vi "tm481_wview_wVision.vi"() -> ()   [LabVIEW 2021]
panel:
  out "Display":T1(plugin-control)
  in  "Vertical Width":i32=512
  in  "Horizontal Width":i32=512
  in  "Vertical Offset B":i32=64
  in  "Horizontal Offset B":i32=256
  in  "Vertical Offset A":i32=128
  in  "Horizontal Offset A":i32=512
  out "Frames Per Second":dbl
  in  "Quit":bool
  out "Error Out":errorcluster {"code" format="%.0x"}
  # "This is just a simple example\nof how to setup a camera for\na W-View application with\na Flash4.0 LT"
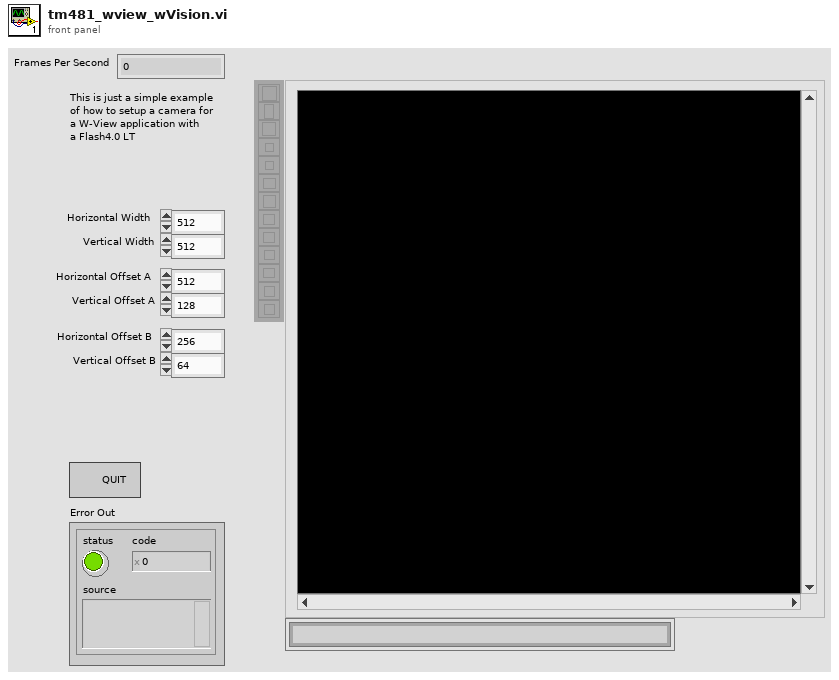
[diagram p1: front panel]
types:
  T1 = typedef "IMAQ Image.ctl" = refnum<image>
  T2 = typedef "Image Type" = u32
  T3 = cluster{"Horizontal Offset A":i32, "Vertical Offset A":i32, "Horizontal Offset B":i32, "Vertical Offset B":i32, "Horizontal Width":i32, "Vertical Width":i32}
  T4 = cluster{"height":i32, "width":i32, "datatype":i32}
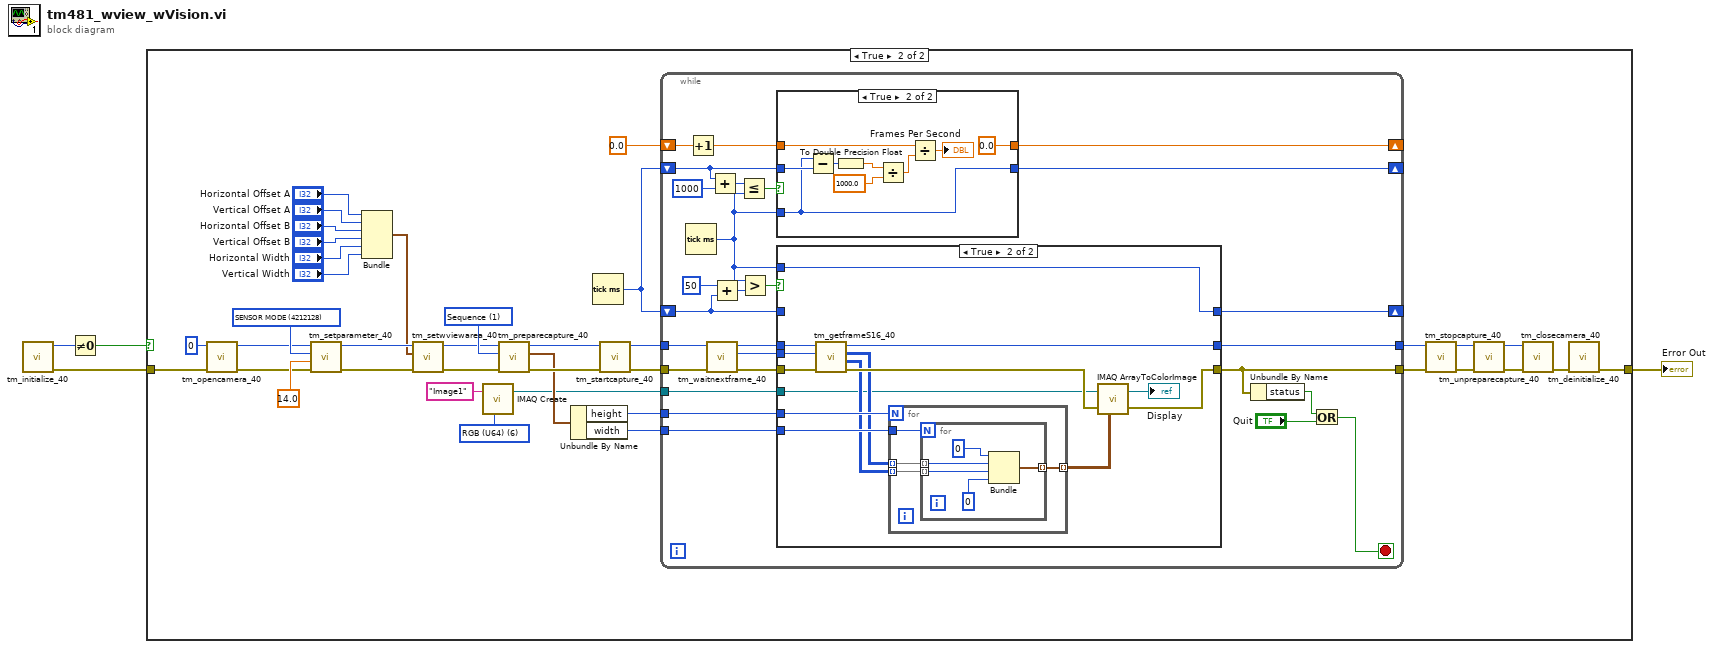
[diagram p0: block diagram]
diagram:
  n1 = call <userlib>:"tm_initialize_40.vi"() -> ("error out"=w1:errorcluster, "Number Of Cameras"=w2:u32)  [unwired: 8 in, 2 out]
  n2 = Not Equal To 0?(x=w2) -> (x != 0?=w4:bool)
  n3 = case shown="True" w4 {
    tunnel: w1 -> [w5 w43]
    tunnel: [w5 w40] -> w3
    frame False {
    }
    frame True {
      w9 = T2 6 items=["Grayscale (U8)", "Grayscale (I16)", "Grayscale (SGL)", "Complex (CSG)", "RGB (U32)", "HSL (U32)", "RGB (U64)", "Grayscale (U16)"] ("Image Type")
      w25 = u32 4212128 items=["SENSOR MODE"=4212128, "CCD MODE"=4212384, "READOUT MODE"=4211872, "ACTIVE VIEW INDEX"=4343136, "BITS PER CHANNEL"=4342976, "IMAGE PIXEL TYPE"=4343296, "BINNING"=4215968, "EXPOSURE TIME"=2049184, "CONTRAST GAIN"=3163312, "CONTRAST OFFSET"=3163328, "LIGHT MODE"=2114720, "SENSITIVITY"=2114992, "PHOTON IMAGING MODE"=2115200, "HIGH DYNAMIC RANGE MODE"=3163360, "WHITE BALANCE"=3163568, "TEMPERATURE"=2115232, "TEMPERATURE TARGET"=2115264, "SENSOR COOLER FAN"=2115296, "LINEBUNDLE HEIGHT"=4212192, "MECHANICAL SHUTTER"=2115488, "BACK FOCUS POSITION"=8422304, "TRIGGER CONNECTOR"=1066432, "TRIGGER SOURCE"=1066144, "OUTPUT TRIGGER SOURCE"=1852576, "TRIGGER GLOBAL EXPOSURE"=2049680, "FIRST TRIGGER BEHAVIOR"=2049696, "CHANNEL SYNC"=1852352, "READOUT DIRECTION"=4211904, "PRE HSYNC COUNT"=1852704, "INTERNAL LINE SPEED"=4191408, "INTERNAL LINE INTERVAL"=4191424] ("Parameter")
      w31 = 1 items=["Snap", "Sequence"] ("Capture mode")
      n4 = call <userlib>:"tm_opencamera_40.vi"("error in (no error)"=w43, "Camera Index"=u32 0) -> ("error out"=w23:errorcluster, "Handle out"=w24:u32)  [unwired: 7 in, 1 out]
      n5 = call <userlib>:"tm_setparameter_40.vi"("error in (no error)"=w23, "Value in"=14.0, "Parameter"=w25, "Handle in"=w24) -> ("error out"=w21:errorcluster, "Handle out"=w22:u32)  [unwired: 6 in]
      n6 = Bundle("Horizontal Offset A"="Horizontal Offset A", "Vertical Offset A"="Vertical Offset A", "Horizontal Offset B"="Horizontal Offset B", "Vertical Offset B"="Vertical Offset B", "Horizontal Width"="Horizontal Width", "Vertical Width"="Vertical Width") -> (w18:T3)  [unwired: 1 in]
      n7 = call <userlib>:"tm_setwviewarea_40.vi"("error in (no error)"=w21, "Sub Region"=w18, "Handle in"=w22) -> ("error out"=w20:errorcluster, "Handle out"=w19:u32)  [unwired: 7 in]
      n8 = call "IMAQ Create"("Image Name"="Image1", "Image Type"=w9) -> ("New Image"=w8:T1)  [unwired: 3 in, 1 out]
      n9 = call <userlib>:"tm_preparecapture_40.vi"("error in (no error)"=w20, "Capture mode"=w31, "Handle in"=w19) -> ("error out"=w29:errorcluster, "Buffer Info"=w11:T4, "Handle out"=w30:u32)  [unwired: 5 in, 1 out]
      n10 = Unbundle By Name(w11) -> ("height"=w7:i32, "width"=w6:i32)
      n11 = Tick Count (ms)() -> (millisecond timer value=w27:u32)
      n12 = call <userlib>:"tm_startcapture_40.vi"("error in (no error)"=w29, "Handle in"=w30) -> ("error out"=w32:errorcluster, "Handle out"=w33:u32)  [unwired: 8 in]
      n13 = while {
        tunnel: [w49] -> w36
        tunnel: [w50] -> w37
        tunnel: w33 -> [w67]
        tunnel: w32 -> [w68]
        shift-right: [w65] -> _
        shift-left: w27 -> [w62]
        shift-right: [w66] -> _
        shift-left: 0.0 -> [w59]
        shift-right: [w48] -> _
        shift-left: w27 -> [w51]
        tunnel: w7 -> [w47]
        tunnel: w6 -> [w46]
        tunnel: w8 -> [w45]
        stop <- w44 stop-if-true
        n14 = Tick Count (ms)() -> (millisecond timer value=w52:u32)
        n15 = Increment(x=w59) -> (x+1=w60:dbl)
        n16 = call <userlib>:"tm_waitnextframe_40.vi"("error in (no error)"=w68, "Handle in"=w67) -> ("error out"=w57:errorcluster, "Frame Index"=w56:i32, "Handle out"=w58:u32)  [unwired: 6 in, 1 out]
        n17 = Add(x=w62, y=u32 1000) -> (x+y=w64:u32)
        n18 = Add(x=u32 50, y=w51) -> (x+y=w54:u32)
        n19 = Less Or Equal?(x=w64, y=w52) -> (x <= y?=w61:bool)
        n20 = Greater?(x=w52, y=w54) -> (0:w53:bool)
        n21 = case shown="True" w61 {
          tunnel: w62 -> [w98 w101]
          tunnel: [w98 w99] -> w65
          tunnel: w60 -> [w97 w105]
          tunnel: w52 -> [_ w99]
          tunnel: [w97 0.0] -> w66
          frame False {
          }
          frame True {
            n22 = Subtract(x=w99, y=w101) -> (x-y=w100:u32)
            n23 = To Double Precision Float(number=w100) -> (double precision float=w107:dbl)
            n24 = Divide(x=w107, y=1000.0) -> (x/y=w104:dbl)
            n25 = Divide(x=w105, y=w104) -> (x/y=→"Frames Per Second":dbl)
          }
        }
        n26 = case shown="True" w53 {
          tunnel: w58 -> [w73 w84]
          tunnel: w57 -> [w72 w86]
          tunnel: w56 -> [_ w85]
          tunnel: w51 -> [w71 _]
          tunnel: w52 -> [_ w87]
          tunnel: [w73 w83] -> w49
          tunnel: [w72 w75] -> w50
          tunnel: [w71 w87] -> w48
          tunnel: w47 -> [_ w81]
          tunnel: w46 -> [_ w80]
          tunnel: w45 -> [_ w74]
          frame False {
          }
          frame True {
            n27 = call <userlib>:"tm_getframeS16_40.vi"("error in (no error)"=w86, "Frame Index"=w85, "Handle in"=w84) -> ("error out"=w82:errorcluster, "Data B"=w78:u16[][], "Data A"=w79:u16[][], "Handle out"=w83:u32)  [unwired: 4 in, 1 out]
            n28 = for {
              N: w81 -> [_]
              tunnel: w80 -> [w91]
              tunnel: w79 -> [w90] mode=indexing
              tunnel: w78 -> [w89] mode=indexing
              tunnel: [w88] -> w77 mode=indexing
              n29 = for {
                N: w91 -> [_]
                tunnel: w90 -> [w94] mode=indexing
                tunnel: w89 -> [w93] mode=indexing
                tunnel: [w95] -> w88 mode=indexing
                n30 = Bundle(u16 0, "Numeric"=w94, "Numeric"=w93, u16 0) -> (w95:cluster{u16, "Numeric":u16, "Numeric":u16, u16})  [unwired: 1 in]
              }
            }
            n31 = call "IMAQ ArrayToColorImage"("Image"=w74, "Image Pixels (U64)"=w77, "error in (no error)"=w82) -> ("Image Out"=→"Display":T1, "error out"=w75:errorcluster)  [unwired: 2 in]
          }
        }
        n32 = Unbundle By Name(w50) -> ("status"=w70:bool)
        n33 = Or(x=w70, y="Quit") -> (x .or. y?=w44:bool)
      }
      n34 = call <userlib>:"tm_stopcapture_40.vi"("error in (no error)"=w37, "Handle in"=w36) -> ("error out"=w34:errorcluster, "Handle out"=w35:u32)  [unwired: 8 in]
      n35 = call <userlib>:"tm_unpreparecapture_40.vi"("error in (no error)"=w34, "Handle in"=w35) -> ("error out"=w39:errorcluster, "Handle out"=w38:u32)  [unwired: 8 in]
      n36 = call <userlib>:"tm_closecamera_40.vi"("error in (no error)"=w39, "Handle in"=w38) -> ("error out"=w41:errorcluster)  [unwired: 9 in]
      n37 = call <userlib>:"tm_deinitialize_40.vi"("error in (no error)"=w41) -> ("error out"=w40:errorcluster)  [unwired: 10 in]
    }
  }
  "Error Out" <- w3
